vi "type change.vi"(10 "Main Vari in":T1={"Error"={"status"=FALSE, "code"=0, "source"=""}, "Test Info"={"Test Name"="", "Tester"=""}, "StateName"="", "Task Info"={"Accele Task"=[], "Simulate"=FALSE, "采样率"={"AISampleRate"=10123, "CouplingType"=10000, "Butter"=1000}, "Trig"={"PreTrigCNT"=0, "TriggerMode"=enum."中间触发", "TriggerSource"=enum."软件触发", "ATRTriggerChannel"=enum."通道0", "TriggerDir"=enum."下降沿触发", "TrigLevelVolt"=0.0, "bAvailableTrig"=FALSE}, "clock"={"EN"=FALSE, "clocksource"=enum."内部时钟", "outclocksource"=enum."Trig0"}, "delay(S)"=0.0}, "Virb Wave"=[{"t0"=timestamp(3350015091.8292503 s since 1904-01-01), "dt"=0.001, "Y"=array[1000 elements], "attributes"=variant("NI_ChannelName"=variant(string "PXI-6221/ai1"), "NI_UnitDescription"=variant(string "Deg C"))}], "Display Info"=[{"Frequency"=0.0, "RMS"=0.0}, {"Frequency"=0.0, "RMS"=0.0}, {"Frequency"=0.0, "RMS"=0.0}, {"Frequency"=0.0, "RMS"=0.0}, {"Frequency"=0.0, "RMS"=0.0}], "粉尘特性"={"名称"="", "粒径"="", "含水量"=""}, "测试条件"={"初始含氧量"="", "初始压力"="", "测试浓度"="", "点火能量"="", "初始温度"="", "反应器体积[L]"=0.0}, "ch size"=0} {"Task Info"."采样率"."CouplingType" items=["直流耦合", "交流耦合"]}) -> (0 "Main Vari out":T1={"Error"={"status"=FALSE, "code"=0, "source"=""}, "Test Info"={"Test Name"="", "Tester"=""}, "StateName"="", "Task Info"={"Accele Task"=[], "Simulate"=FALSE, "采样率"={"AISampleRate"=10123, "CouplingType"=10000, "Butter"=1000}, "Trig"={"PreTrigCNT"=0, "TriggerMode"=enum."中间触发", "TriggerSource"=enum."软件触发", "ATRTriggerChannel"=enum."通道0", "TriggerDir"=enum."下降沿触发", "TrigLevelVolt"=0.0, "bAvailableTrig"=FALSE}, "clock"={"EN"=FALSE, "clocksource"=enum."内部时钟", "outclocksource"=enum."Trig0"}, "delay(S)"=0.0}, "Virb Wave"=[{"t0"=timestamp(3350015091.8292503 s since 1904-01-01), "dt"=0.001, "Y"=array[1000 elements], "attributes"=variant("NI_ChannelName"=variant(string "PXI-6221/ai1"), "NI_UnitDescription"=variant(string "Deg C"))}], "Display Info"=[{"Frequency"=0.0, "RMS"=0.0}, {"Frequency"=0.0, "RMS"=0.0}, {"Frequency"=0.0, "RMS"=0.0}, {"Frequency"=0.0, "RMS"=0.0}, {"Frequency"=0.0, "RMS"=0.0}], "粉尘特性"={"名称"="", "粒径"="", "含水量"=""}, "测试条件"={"初始含氧量"="", "初始压力"="", "测试浓度"="", "点火能量"="", "初始温度"="", "反应器体积[L]"=0.0}, "ch size"=0} {"Task Info"."采样率"."CouplingType" items=["直流耦合", "交流耦合"]}, 1 "set para":T10={"buffer size"=524288, "pci 8532 para"={"Ch"=[1, 1, 1, 1], "inputrange"=[1, 1, 1, 1], "采样频率"=10000, "耦合类型"=1, "预置触发计数器"=1024, "触发模式选择"=0, "ART通道选择"=0, "触发源"=0, "触发方向"=0, "当触发提前时，是否有效"=0, "时钟源"=0, "时钟输入输出源"=0, "是否将时钟信号输入到同步总线"=1}, "segment"={"nReadSizeWords"=8192, "nSegmentCount"=64, "nSegmentSizeWords"=8192}})   [LabVIEW 2011]
uses:
  Ctrls/Main vari.ctl
  Ctrls/Task Info.ctl
  Ctrls/Sample Information.ctl
  Ctrls/Trig.ctl
  Ctrls/clock.ctl
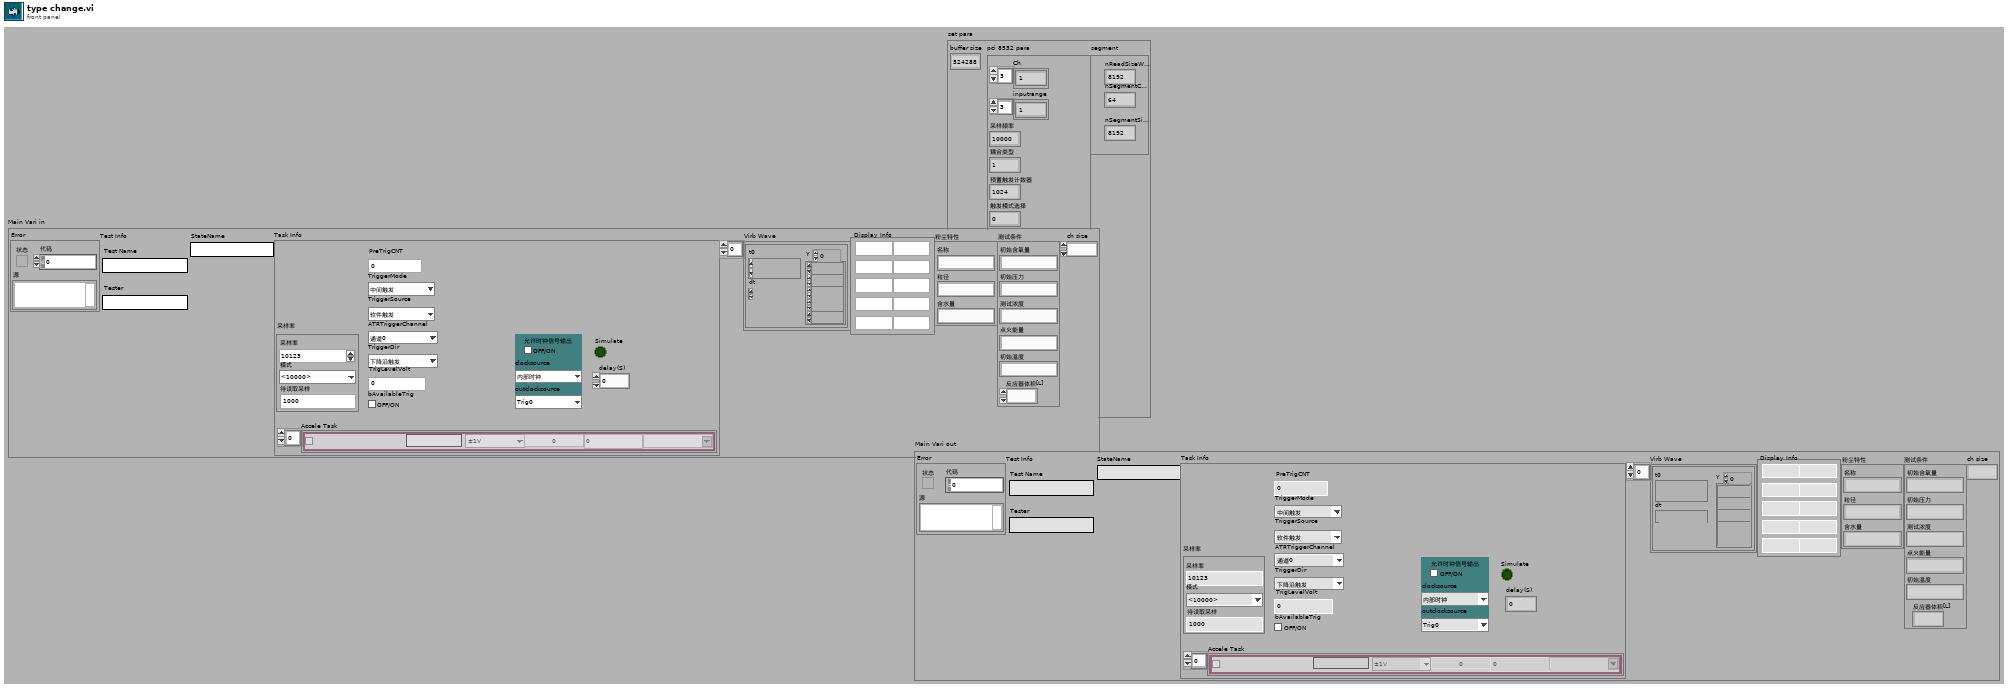
[diagram p1: front panel]
types:
  T1 = typedef "Main vari.ctl" = cluster{"Error":errorcluster, "Test Info":cluster{"Test Name":string, "Tester":string}, "StateName":string, "Task Info":T2, "Virb Wave":waveform(dbl)[], "Display Info":T7, "粉尘特性":T8, "测试条件":T9, "ch size":u8}
  T2 = typedef "Task Info.ctl" = cluster{"Accele Task":T3[], "Simulate":bool, "采样率":T4, "Trig":T5, "clock":T6, "delay(S)":dbl}
  T3 = typedef "Acceleration Channel Config_Ctrls-某型振动实验台测试系统.ctl" = cluster{"Enable":bool, "Name":string, "range":enum16{"±1V", "±5V"}, "SensValue":dbl, "PhysicalName":string, "off":dbl, "Sensunits":string}
  T4 = typedef "Sample Information.ctl" = cluster{"AISampleRate":i32, "CouplingType":i32, "Butter":i32}
  T5 = typedef "Trig.ctl" = cluster{"PreTrigCNT":i32, "TriggerMode":enum16{"中间触发", "后触发", "预触发", "硬件延时触发"}, "TriggerSource":enum16{"软件触发", "DTR信号源", "ATR信号源", "Triger信号触发"}, "ATRTriggerChannel":enum16{"通道0", "通道1", "通道2", "通道3"}, "TriggerDir":enum16{"下降沿触发", "上升沿触发", "上下边没均触发"}, "TrigLevelVolt":sgl, "bAvailableTrig":bool}
  T6 = typedef "clock.ctl" = cluster{"EN":bool, "clocksource":enum16{"内部时钟", "外部时钟"}, "outclocksource":enum16{"Trig0", "Trig1", "Trig2", "Trig3", "Trig4", "Trig5", "Trig6", "Trig7", "PXI_STAR"}}
  T7 = typedef "Display Information_Ctrls-某型振动实验台测试系统.ctl" = cluster{"Frequency":dbl, "RMS":dbl}[]
  T8 = typedef "粉尘特性.ctl" = cluster{"名称":string, "粒径":string, "含水量":string}
  T9 = typedef "测试条件.ctl" = cluster{"初始含氧量":string, "初始压力":string, "测试浓度":string, "点火能量":string, "初始温度":string, "反应器体积[L]":dbl}
  T10 = cluster{"buffer size":i32, "pci 8532 para":cluster{"Ch":i32[], "inputrange":i32[], "采样频率":i32, "耦合类型":i32, "预置触发计数器":i32, "触发模式选择":i32, "ART通道选择":i32, "触发源":i32, "触发方向":i32, "当触发提前时，是否有效":i32, "时钟源":i32, "时钟输入输出源":i32, "是否将时钟信号输入到同步总线":i32}, "segment":cluster{"nReadSizeWords":i32, "nSegmentCount":i32, "nSegmentSizeWords":i32}}
  T11 = enum16{"Trig0", "Trig1", "Trig2", "Trig3", "Trig4", "Trig5", "Trig6", "Trig7", "PXI_STAR"}
  T12 = cluster{"nReadSizeWords":i32, "nSegmentCount":i32, "nSegmentSizeWords":i32}
  T13 = cluster{"Ch":i32[], "inputrange":i32[], "采样频率":i32, "耦合类型":i32, "预置触发计数器":i32, "触发模式选择":i32, "ART通道选择":i32, "触发源":i32, "触发方向":i32, "当触发提前时，是否有效":i32, "时钟源":i32, "时钟输入输出源":i32, "是否将时钟信号输入到同步总线":i32}
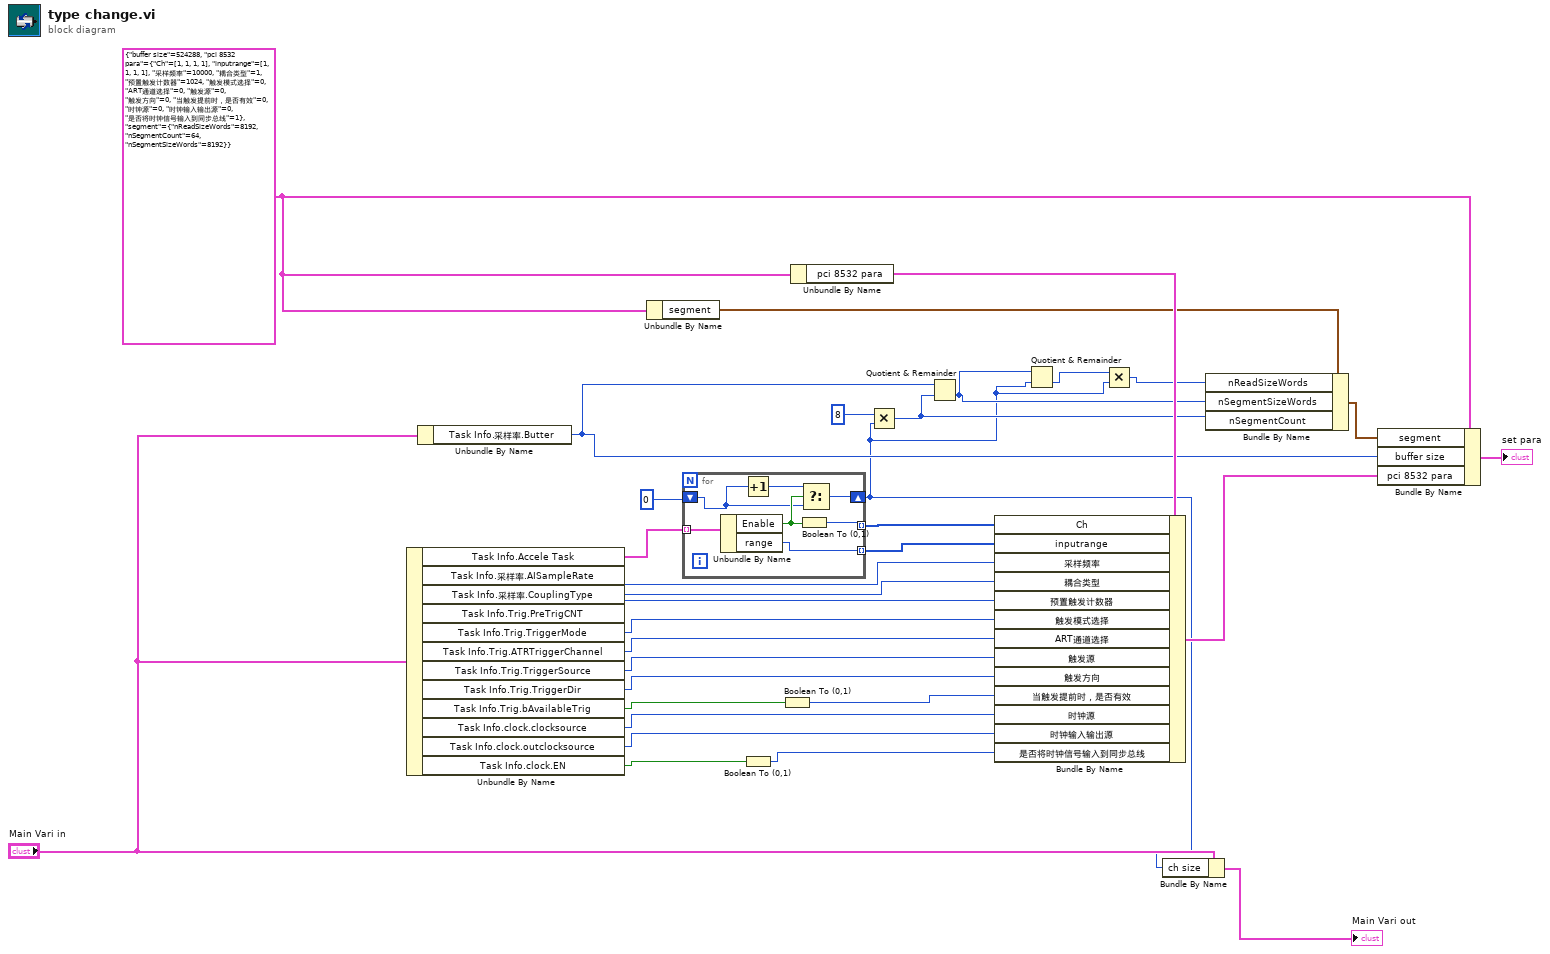
[diagram p0: block diagram]
diagram:
  w13 = T10 {"buffer size"=524288, "pci 8532 para"={"Ch"=[1, 1, 1, 1], "inputrange"=[1, 1, 1, 1], "采样频率"=10000, "耦合类型"=1, "预置触发计数器"=1024, "触发模式选择"=0, "ART通道选择"=0, "触发源"=0, "触发方向"=0, "当触发提前时，是否有效"=0, "时钟源"=0, "时钟输入输出源"=0, "是否将时钟信号输入到同步总线"=1}, "segment"={"nReadSizeWords"=8192, "nSegmentCount"=64, "nSegmentSizeWords"=8192}} ("set para")
  n1 = Unbundle By Name("Main Vari in") -> ("Task Info.Accele Task"=w29:T3[], "Task Info.采样率.AISampleRate"=w26:i32, "Task Info.采样率.CouplingType"=w25:i32, "Task Info.Trig.PreTrigCNT"=w24:i32, "Task Info.Trig.TriggerMode"=w23:enum16{"中间触发", "后触发", "预触发", "硬件延时触发"}, "Task Info.Trig.ATRTriggerChannel"=w22:enum16{"通道0", "通道1", "通道2", "通道3"}, "Task Info.Trig.TriggerSource"=w21:enum16{"软件触发", "DTR信号源", "ATR信号源", "Triger信号触发"}, "Task Info.Trig.TriggerDir"=w20:enum16{"下降沿触发", "上升沿触发", "上下边没均触发"}, "Task Info.Trig.bAvailableTrig"=w19:bool, "Task Info.clock.clocksource"=w17:enum16{"内部时钟", "外部时钟"}, "Task Info.clock.outclocksource"=w16:T11, "Task Info.clock.EN"=w15:bool)
  n2 = Unbundle By Name("Main Vari in") -> ("Task Info.采样率.Butter"=w9:i32)
  n3 = Unbundle By Name(w13) -> ("segment"=w12:T12)
  n4 = for {
    tunnel: w29 -> [w39] mode=indexing
    tunnel: [w37] -> w28 mode=indexing
    tunnel: [w38] -> w27 mode=indexing
    shift-right: [w33] -> w1
    shift-left: 0 -> [w35]
    n5 = Unbundle By Name(w39) -> ("Enable"=w36:bool, "range"=w38:enum16{"±1V", "±5V"})
    n6 = Increment(x=w35) -> (x+1=w34:i32)
    n7 = Boolean To (0,1)(Boolean=w36) -> (0, 1=w37:i16)
    n8 = Select(t=w34, s=w36, f=w35) -> (s? t:f=w33:i32)
  }
  n9 = Boolean To (0,1)(Boolean=w15) -> (0, 1=w14:i16)
  n10 = Boolean To (0,1)(Boolean=w19) -> (0, 1=w18:i16)
  n11 = Unbundle By Name(w13) -> ("pci 8532 para"=w31:T13)
  n12 = Multiply(x=8, y=w1) -> (x*y=w7:i32)
  n13 = Quotient & Remainder(x=w9, y=w7) -> (floor(x/y)=w6:i32)  [unwired: 1 out]
  n14 = Bundle By Name(cluster=w31, "Ch"=w28, "inputrange"=w27, "采样频率"=w26, "耦合类型"=w25, "预置触发计数器"=w24, "触发模式选择"=w23, "ART通道选择"=w22, "触发源"=w21, "触发方向"=w20, "当触发提前时，是否有效"=w18, "时钟源"=w17, "时钟输入输出源"=w16, "是否将时钟信号输入到同步总线"=w14) -> (w30:T13)
  n15 = Quotient & Remainder(x=w6, y=w1) -> (floor(x/y)=w5:i32)  [unwired: 1 out]
  n16 = Multiply(x=w5, y=w1) -> (x*y=w4:i32)
  n17 = Bundle By Name(cluster="Main Vari in", "ch size"=w1) -> (→"Main Vari out":T1)
  n18 = Bundle By Name(cluster=w12, "nReadSizeWords"=w4, "nSegmentSizeWords"=w6, "nSegmentCount"=w7) -> (w10:T12)
  n19 = Bundle By Name(cluster=w13, "segment"=w10, "buffer size"=w9, "pci 8532 para"=w30) -> (→"set para":T10)
